vi "Configure Width Trigger Source [WT].vi"(0 "CS++Scope":refnum<class "CS++Scope.lvclass">, 1 "trigger source (\"CHANNEL1\")":string(combo)="CHANNEL1", 2 "trigger level (0.0 V)":dbl[unit] format="%.3f", 3 "width condition (Within)":i32(ring)=1 items=["Within"=1, "Outside"=2], 4 "width polarity (Positive)":i32(ring)=1 items=["Positive"=1, "Negative"=2], 5 "error in (no error)":errorcluster, 6 "width low threshold (1.0 E-9 V)":dbl[unit]=1e-09 format="%^.3e", 8 "width high threshold (2.0 E-9 V)":dbl[unit]=2e-09 format="%^.3e") -> (14 "CS++Scope out":refnum<class "CS++Scope.lvclass">, 19 "error out":errorcluster)   [LabVIEW 2013, in "CS++Scope.lvlib" / "CS++Scope.lvclass"]
doc: "This VI configures the width trigger. A width trigger occurs when the oscilloscope detects a positive or negative pulse with a width between, or optionally outside, the width thresholds. You specify the width thresholds with the Width Low Threshold and Width High Threshold parameters. You specify whether the oscilloscope triggers on pulse widths that are within or outside the width thresholds with the Width Condition parameter. You specify the polarity of the pulse with the Width Polarity parameter. The trigger does not actually occur until the edge of a pulse that corresponds to the Width Low Threshold, Width High Threshold, Width Condition, and Width Polarity crosses the threshold you specify in the Trigger Level parameter.\n\nNote (1) This VI affects instrument behavior only if the trigger type is IVISCOPE_VAL_WIDTH_TRIGGER. Call the IviScope Configure Trigger and IviScope Configure Trigger Coupling VIs to set the trigger type and trigger coupling before calling this VI.\n(2) This VI is part of the IviScopeWidthTrigger [WT] extension group."
uses:
  CS++Scope.lvclass
  CSPP_Core/Classes/CS++ProcessVariables/ProcessVariable/PV.lvclass
  PV-Enum.ctl
  CS++Scope.lvclass/CS++Scope.ctl
  CSPP_Core/Classes/CS++ProcessVariables/PVConnection/PVConnection.lvclass
  CSPP_Core/Classes/CS++ProcessVariables/ProcessVariable/PV.lvclass/PV.ctl
  CSPP_Core/Classes/CS++ProcessVariables/ProcessVariable/Write Data.vi
  CSPP_Core/Classes/CS++ProcessVariables/ProcessVariable/Write Timestamp.vi
  CSPP_Core/Classes/CS++ProcessVariables/ProcessVariable/Write Quality.vi
  CSPP_Core/Classes/CS++ProcessVariables/ProcessVariable/Write status.vi
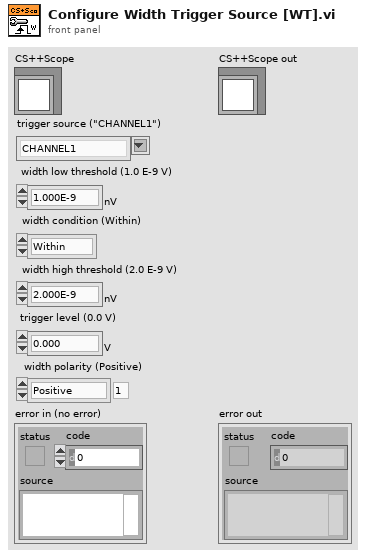
[diagram p1: front panel]
types:
  T1 = typedef "CS++Scope.lvlib/CS++Scope.lvclass/PV-Enum.ctl" = enum16{"ActualSampleRate", "TimePerRecord", "AcquisitionStartTime", "TriggerLevel", "GlitchWidth", "LowReference", "MidReference", "HighReference", "RuntLowThreshold", "RuntHighThreshold", "TriggerHoldoff", "WidthLowThreshold", "WidthHighThreshold", "AcquisitionStatus", "ActualRecordLength", "ActualSampleMode", "ACLineTriggerSlope", "MinRecordLength", "AcquisitionType", "TriggerSlope", "GlitchCondition", "GlitchPolarity", "InterpolationMethod", "NumberOfAverages", "NumberOfEnvelopes", "TriggerType", "TriggerCoupling", "TriggerModifier", "TVLineNumber", "TVEvent", "TVTriggerPolarity", "TVSignalFormat", "WidthCondition", "WidthPolarity", "MeasurementDone", "ContinousAcquisition", "TriggerSource", "Waveform"}
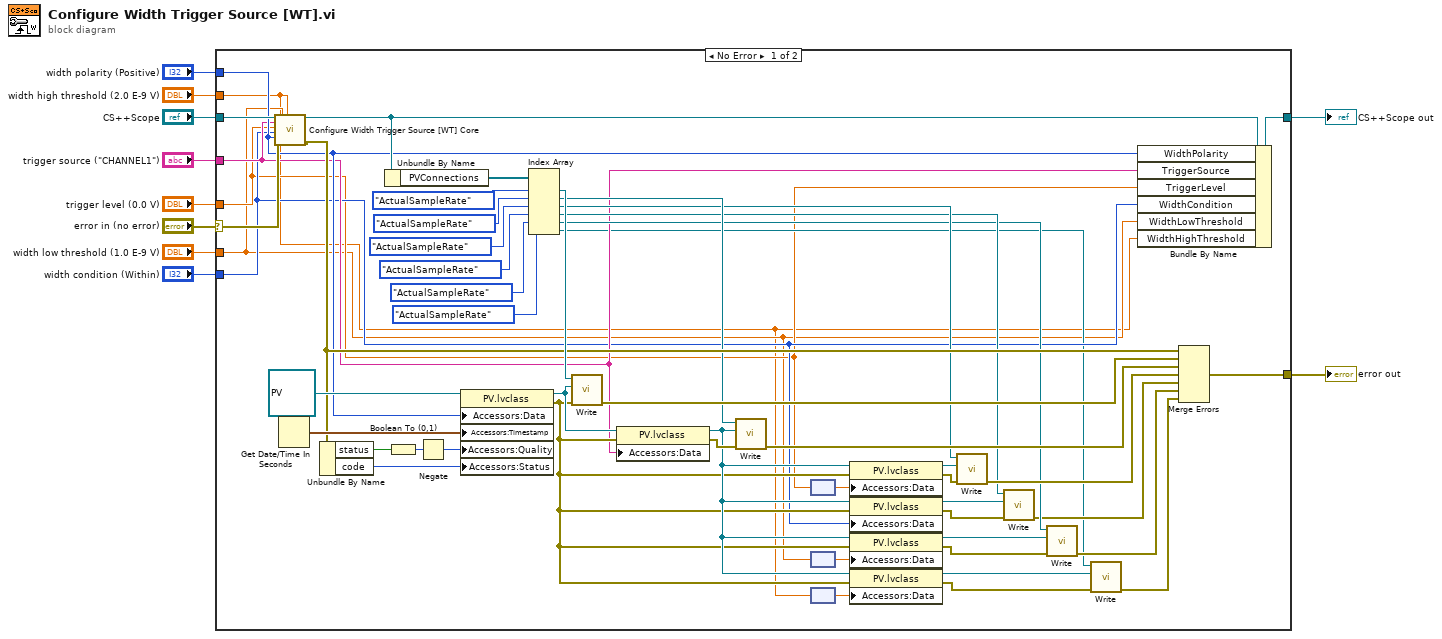
[diagram p0: block diagram]
diagram:
  n1 = case shown="No Error" "error in (no error)" {
    selector: "error in (no error)" -> [w28 w64]
    tunnel: [w27 w64] -> w9
    tunnel: [w29 w63] -> w1
    tunnel: "CS++Scope" -> [w30 w63]
    tunnel: "trigger source (\"CHANNEL1\")" -> [w20 _]
    tunnel: "trigger level (0.0 V)" -> [w16 _]
    tunnel: "width low threshold (1.0 E-9 V)" -> [w14 _]
    tunnel: "width condition (Within)" -> [w19 _]
    tunnel: "width high threshold (2.0 E-9 V)" -> [w12 _]
    tunnel: "width polarity (Positive)" -> [w21 _]
    frame No Error {
      n2 = call-dynamic "Configure Width Trigger Source [WT] Core.vi"("CS++Scope"=w30, "trigger source (\"CHANNEL1\")"=w20, "trigger level (0.0 V)"=w16, "width condition (Within)"=w19, "width polarity (Positive)"=w21, "error in (no error)"=w28, "width low threshold (1.0 E-9 V)"=w14, "width high threshold (2.0 E-9 V)"=w12) -> ("CS++Scope out"=w52:refnum<class "CS++Scope.lvclass">, "error out"=w51:errorcluster)  [unwired: 10 in]
      n3 = Get Date/Time In Seconds() -> (seconds since 1Jan1904=w57:timestamp)
      n4 = Unbundle By Name(w51) -> ("status"=w60:bool, "code"=w61:i32)
      n5 = Unbundle By Name(w52) -> ("PVConnections"=w56:refnum<class "PVConnection.lvclass">[])
      n6 = Boolean To (0,1)(Boolean=w60) -> (0, 1=w59:i16)
      n7 = Negate(x=w59) -> (-x=w58:i16)
      n8 = property class="PV.lvclass"(reference=refnum<class "PV.lvclass"> refnum ("CS++ProcessVariables.lvlib:PV.lvclass"), "Accessors:Data"=w21, "Accessors:Timestamp"=w57, "Accessors:Quality"=w58, "Accessors:Status"=w61) -> (reference out=w46:refnum<class "PV.lvclass">, error out=w25:errorcluster)  [unwired: 1 in]
      n9 = Index Array(array=w56, index #1=PV-Enum."ActualSampleRate" ("PV-Enum"), index #2=PV-Enum."ActualSampleRate" ("PV-Enum"), index #3=PV-Enum."ActualSampleRate" ("PV-Enum"), index #4=PV-Enum."ActualSampleRate" ("PV-Enum"), index #5=PV-Enum."ActualSampleRate" ("PV-Enum"), index #6=PV-Enum."ActualSampleRate" ("PV-Enum")) -> (element #1=w54:refnum<class "PVConnection.lvclass">, element #2=w44:refnum<class "PVConnection.lvclass">, element #3=w42:refnum<class "PVConnection.lvclass">, element #4=w34:refnum<class "PVConnection.lvclass">, element #5=w33:refnum<class "PVConnection.lvclass">, element #6=w18:refnum<class "PVConnection.lvclass">)
      n10 = call-dynamic "Write.vi"("error in (no error)"=w25, "PV"=w46, "PVConnection in"=w54) -> ("error out"=w53:errorcluster)  [unwired: 7 in, 1 out]
      n11 = property class="PV.lvclass"(reference=w46, error in=w25, "Accessors:Data"=w20) -> (reference out=w26:refnum<class "PV.lvclass">, error out=w45:errorcluster)
      n12 = call-dynamic "Write.vi"("error in (no error)"=w45, "PV"=w26, "PVConnection in"=w44) -> ("error out"=w48:errorcluster)  [unwired: 7 in, 1 out]
      n13 = node(w16) -> (w15:dbl)
      n14 = node(w14) -> (w13:dbl)
      n15 = node(w12) -> (w11:dbl)
      n16 = property class="PV.lvclass"(reference=w26, error in=w25, "Accessors:Data"=w15) -> (reference out=w43:refnum<class "PV.lvclass">, error out=w41:errorcluster)
      n17 = property class="PV.lvclass"(reference=w26, error in=w25, "Accessors:Data"=w19) -> (reference out=w38:refnum<class "PV.lvclass">, error out=w37:errorcluster)
      n18 = property class="PV.lvclass"(reference=w26, error in=w25, "Accessors:Data"=w13) -> (reference out=w36:refnum<class "PV.lvclass">, error out=w35:errorcluster)
      n19 = property class="PV.lvclass"(reference=w26, error in=w25, "Accessors:Data"=w11) -> (reference out=w24:refnum<class "PV.lvclass">, error out=w23:errorcluster)
      n20 = call-dynamic "Write.vi"("error in (no error)"=w41, "PV"=w43, "PVConnection in"=w42) -> ("error out"=w47:errorcluster)  [unwired: 7 in, 1 out]
      n21 = call-dynamic "Write.vi"("error in (no error)"=w37, "PV"=w38, "PVConnection in"=w34) -> ("error out"=w32:errorcluster)  [unwired: 7 in, 1 out]
      n22 = call-dynamic "Write.vi"("error in (no error)"=w35, "PV"=w36, "PVConnection in"=w33) -> ("error out"=w31:errorcluster)  [unwired: 7 in, 1 out]
      n23 = call-dynamic "Write.vi"("error in (no error)"=w23, "PV"=w24, "PVConnection in"=w18) -> ("error out"=w22:errorcluster)  [unwired: 7 in, 1 out]
      n24 = Bundle By Name(cluster=w52, "WidthPolarity"=w21, "TriggerSource"=w20, "TriggerLevel"=w16, "WidthCondition"=w19, "WidthLowThreshold"=w14, "WidthHighThreshold"=w12) -> (w29:refnum<class "CS++Scope.lvclass">)
      n25 = Merge Errors(w51, w53, w48, w47, w32, w31, w22) -> (w27:errorcluster)
    }
    frame Error {
    }
  }
  "error out" <- w9
  "CS++Scope out" <- w1
